vi "Negate 00.vi"(1 "x":sgl) -> (0 "-x":sgl)   [LabVIEW 2017]
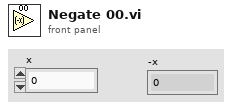
[diagram p1: front panel]
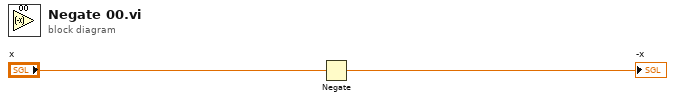
[diagram p0: block diagram]
diagram:
  n1 = Negate(x="x") -> (-x=→"-x":sgl)
